vi "Correct Non-Uniformity.vi"(8 "Error In":errorcluster, 11 "reference in":refnum<class "Flir A700.lvclass">) -> (0 "Error Out":errorcluster, 3 "reference out":refnum<class "Flir A700.lvclass">)   [LabVIEW 2025, in "Flir A700.lvclass"]
uses:
  Flir A700.lvclass
  <vilib>/userDefined/High Color/IMAQdx.ctl
  <resource>/objmgr/imaqdx.rc
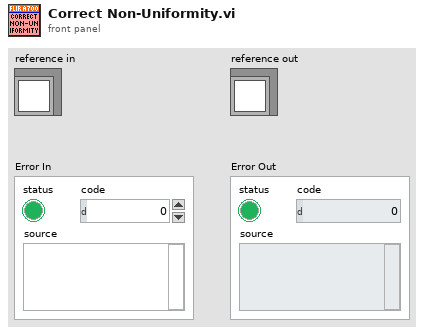
[diagram p1: front panel]
types:
  T1 = typedef "IMAQdx.ctl" = refnum<k21>
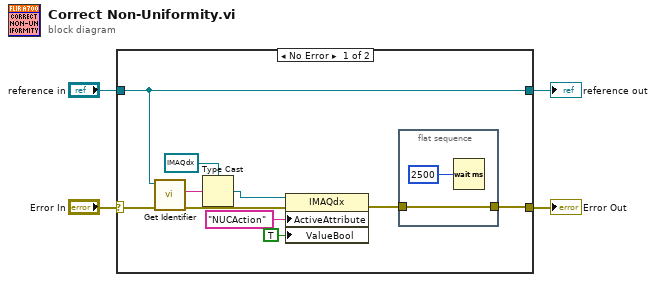
[diagram p0: block diagram]
diagram:
  n1 = case shown="No Error" "Error In" {
    selector: "Error In" -> [w13 w18]
    tunnel: [w5 w18] -> w3
    tunnel: [w14 w17] -> w1
    tunnel: "reference in" -> [w14 w17]
    frame No Error {
      n2 = call-dynamic "Get Identifier.vi"("Error In"=w13, "reference in"=w14) -> ("Error Out"=w12:errorcluster, "Identifier"=w11:string)  [unwired: 7 in, 1 out]
      n3 = Type Cast(type=T1 refnum ("IMAQdx Session"), x=w11) -> (*(type *) &x=w9:T1)
      n4 = property class="IMAQdx"(reference=w9, error in=w12, "ActiveAttribute"="NUCAction", "ValueBool"=TRUE) -> (error out=w6:errorcluster)  [unwired: 1 out]
      n5 = flat-sequence {
        tunnel: w6 -> [w16]
        tunnel: [w16] -> w5
        frame #0 {
          n6 = Wait (ms)(milliseconds to wait=u32 2500) -> ()  [unwired: 1 out]
        }
      }
    }
    frame Error {
    }
  }
  "Error Out" <- w3
  "reference out" <- w1
